vi "ConvertPixelType.vi"(0 "handle":u64, 5 "pSrcData":u8[](array[numeric]), 7 "pDstBuf In":u8[](array[numeric]), 9 "pConvertInfo In":T1, 11 "error in (no error)":errorcluster caption="错误输入（无错误）") -> (4 "handle out":u64, 6 "function return":i32, 8 "pDstBuf Out":u8[](array[numeric]), 10 "pConvertInfo Out":T1, 15 "error out":errorcluster caption="错误输出")   [LabVIEW 2011, in "MvCameraControl.lvlib"]
doc: "MV_CAMPAT_API int __stdcall MV_CP_ConvertPixelType();"
uses:
  MvCameraControl.lvlib
  x86/MvCameraPatch.dll
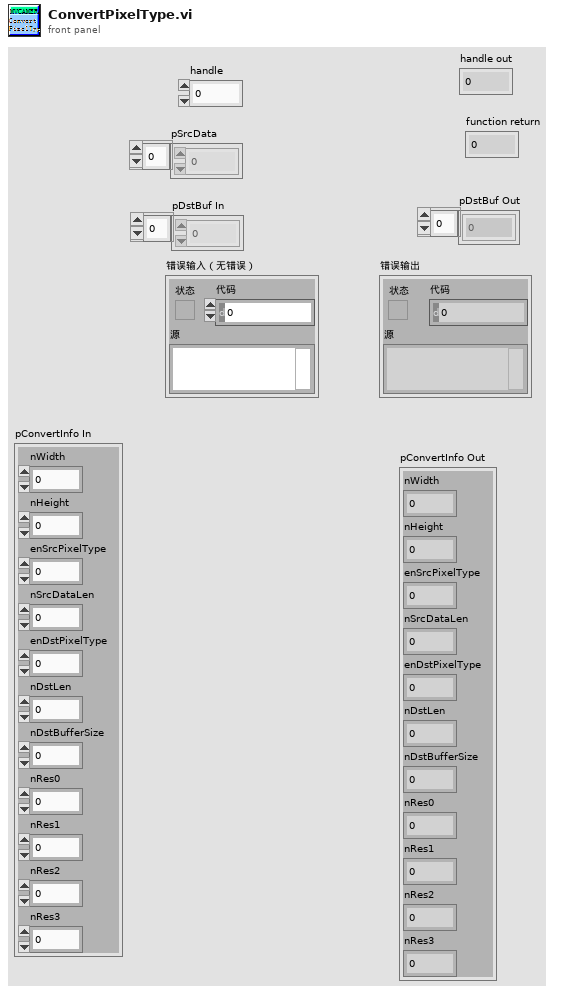
[diagram p1: front panel]
types:
  T1 = cluster{"nWidth":u16, "nHeight":u16, "enSrcPixelType":u32, "nSrcDataLen":u32, "enDstPixelType":u32, "nDstLen":u32, "nDstBufferSize":u32, "nRes0":u32, "nRes1":u32, "nRes2":u32, "nRes3":u32}
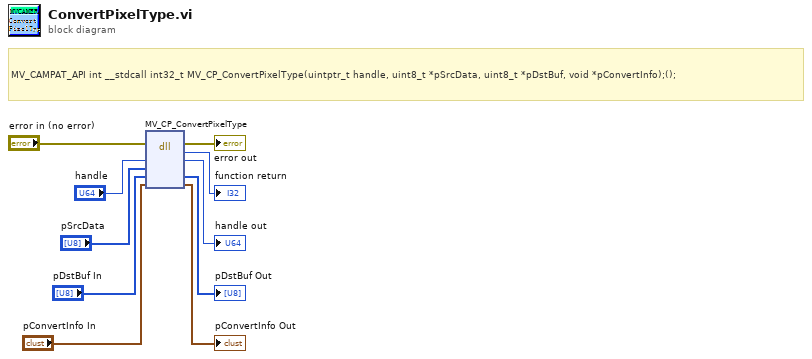
[diagram p0: block diagram]
diagram:
  # "MV_CAMPAT_API int __stdcall int32_t MV_CP_ConvertPixelType(uintptr_t handle, uint8_t *pSrcData, uint8_t *pDstBuf, void *pConvertInfo);();"
  n1 = dll-call lib="F:/SVN/SDK/Release/MVS/Samples/Labview/MvLVLib/x86/MvCameraPatch.dll" fn="MV_CP_ConvertPixelType"(error in="error in (no error)", "handle"="handle", "pSrcData"="pSrcData", "pDstBuf"="pDstBuf In", "pConvertInfo"="pConvertInfo In") -> (error out=→"error out":errorcluster, "返回类型"=→"function return":i32, "handle"=→"handle out":u64, "pDstBuf"=→"pDstBuf Out":u8[], "pConvertInfo"=→"pConvertInfo Out":T1)  [unwired: 3 in, 1 out]
